vi "Subset.vi"   [LabVIEW 2019, in "xy_utilities.lvlib"]
doc: "Returns a subset of the data.\n\nWire data to the data input to determine the polymorphic instance to use or manually select the instance."
uses:
  xy_utilities.lvlib
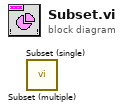
[diagram p0: block diagram]
diagram:
  n1 = call "Subset (multiple).vi"() -> ()  [unwired: 10 in, 2 out]
  n2 = call "Subset (single).vi"() -> ()  [unwired: 10 in, 2 out]
